vi "GymkhanaMonitoring.vi"() -> ()   [LabVIEW 2017]
uses:
  Control/GymkhanaBestIndicator(Monitoring).ctl
  Control/GymkhanaIndicator(Monitoring).ctl
  Control/GymkhanaData.ctl
panel:
  out "CurrentRecordIndicator":T1
  out "BestRecordIndicator":T2
  in  "Stop Button":bool
  # "2018 KSAE Formula Gymkhana Event"
  # "Time :"
  # "Time :"
  # "Entry :"
  # "Entry :"
  # "Univ. :"
  # "Univ. :"
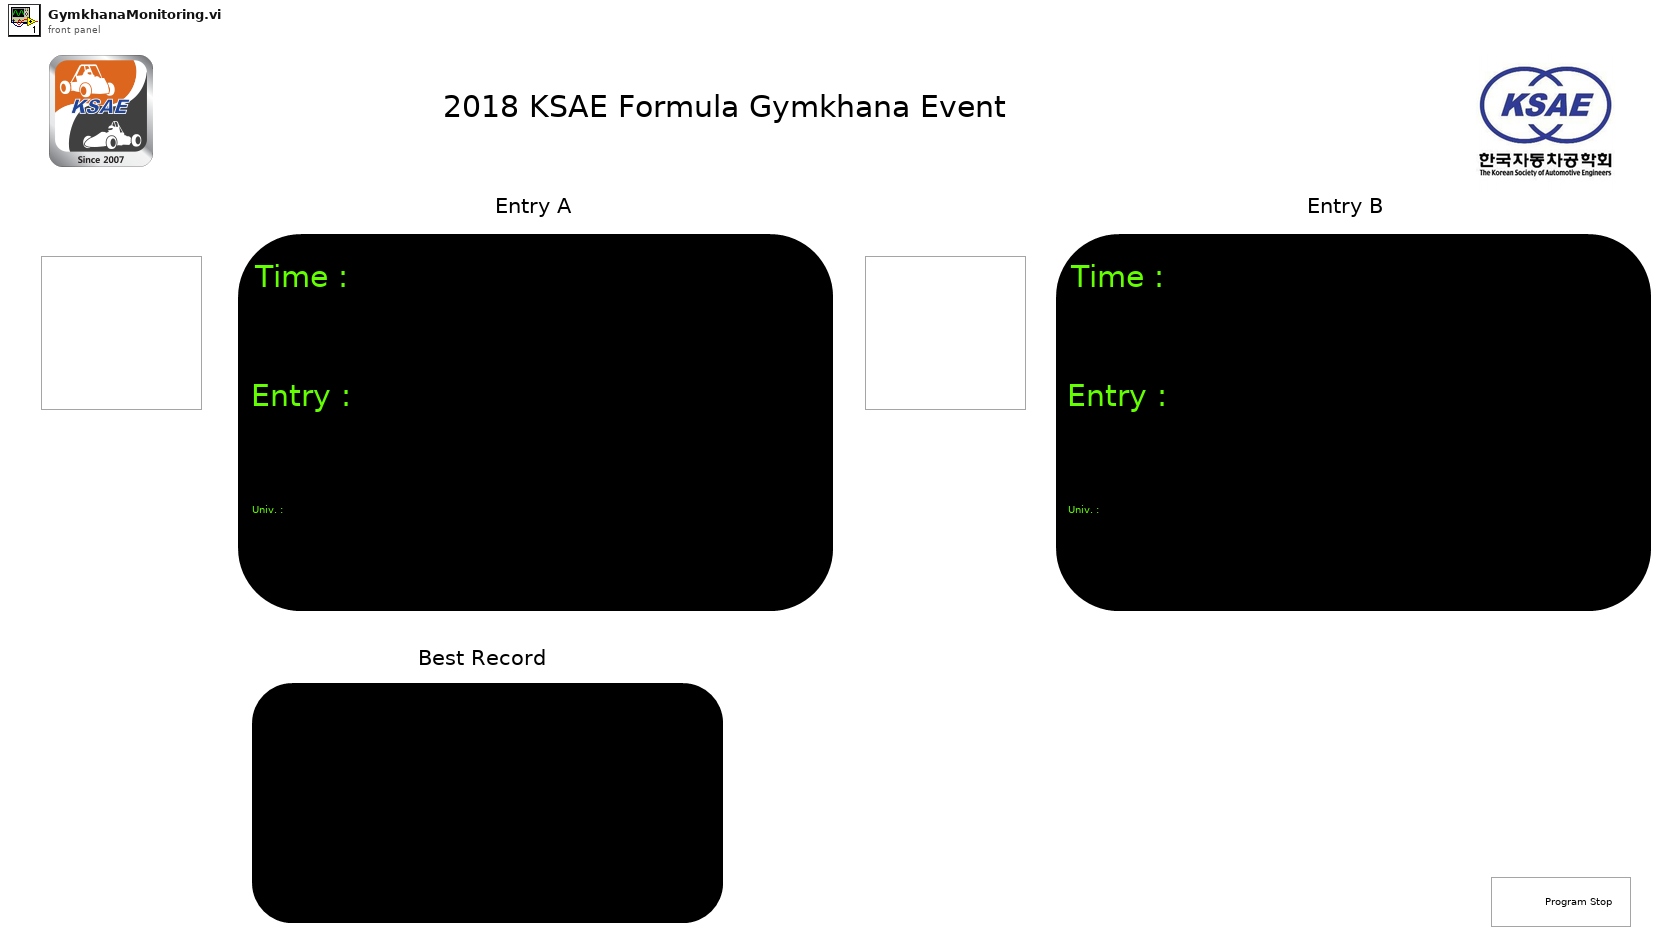
[diagram p1: front panel]
types:
  T1 = typedef "GymkhanaIndicator(Monitoring).ctl" = cluster{"CurrentTime-A":string, "CurrentEntry-A":string, "CurrentUniversity-A":string, "Flag-A":picture, "CurrentMessage-A":string, "CurrentTime-B":string, "CurrentEntry-B":string, "CurrentUniversity-B":string, "Flag-B":picture, "CurrentMessage-B":string}
  T2 = typedef "GymkhanaBestIndicator(Monitoring).ctl" = cluster{"BestTime":string, "BestEntry":string, "BestSchool":string}
  T3 = typedef "GymkhanaData.ctl" = cluster{"LabTime-A":string, "Entry-A":string, "University-A":string, "Flag-A":picture, "Message-A":string, "LabTime-B":string, "Entry-B":string, "University-B":string, "Flag-B":picture, "Message-B":string, "LabTime-Best":string, "Entry-Best":string, "University-Best":string}
  T4 = cluster{"Read Access":enum8{"Allowed", "Required", "None"}, "Write Access":enum8{"Allowed", "Required", "None"}}
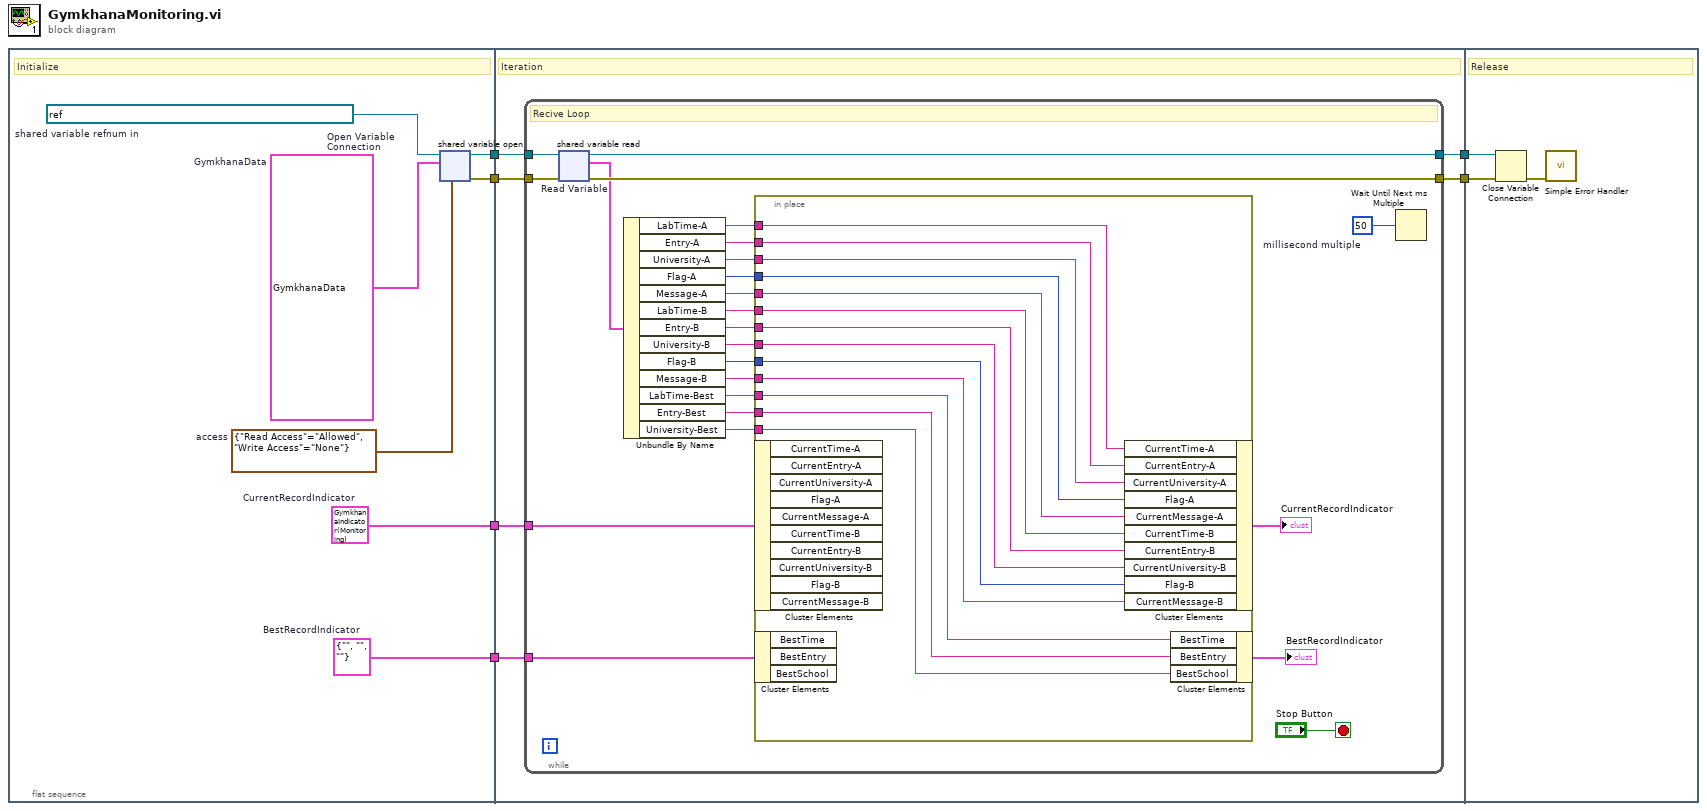
[diagram p0: block diagram]
diagram:
  n1 = flat-sequence {
    tunnel: [w13] -> w6
    tunnel: [w11] -> w5
    tunnel: [w8] -> w2
    tunnel: [w7] -> w1
    tunnel: w6 -> [w19]
    tunnel: w5 -> [w18]
    tunnel: [w17] -> w4
    tunnel: [w16] -> w3
    tunnel: w2 -> [w15]
    tunnel: w1 -> [w14]
    tunnel: w4 -> [w59]
    tunnel: w3 -> [w58]
    frame #0 {
      w7 = T2 {"BestTime"="", "BestEntry"="", "BestSchool"=""}  # BestRecordIndicator
      w8 = T1 {"CurrentTime-A"="", "CurrentEntry-A"="", "CurrentUniversity-A"="", "Flag-A"=bytes[0], "CurrentMessage-A"="", "CurrentTime-B"="", "CurrentEntry-B"="", "CurrentUniversity-B"="", "Flag-B"=bytes[0], "CurrentMessage-B"=""}  # CurrentRecordIndicator
      w9 = T3 {"LabTime-A"="", "Entry-A"="", "University-A"="", "Flag-A"=bytes[0], "Message-A"="", "LabTime-B"="", "Entry-B"="", "University-B"="", "Flag-B"=bytes[0], "Message-B"="", "LabTime-Best"="", "Entry-Best"="", "University-Best"=""}  # GymkhanaData
      w10 = refnum<k21> "ni.var.psp://kdh/MonitoringVariable/GymkhanaData"  # shared variable refnum in
      w12 = T4 {"Read Access"=enum."Allowed", "Write Access"=enum."None"}  # access
      # "Initialize"
      n2 = shared-variable-open "Open Variable Connection"(w10, w9, w12) -> (w13:refnum<k21>, w11:errorcluster)  [unwired: 1 in]
    }
    frame #1 {
      # "Iteration"
      n3 = while {
        tunnel: w19 -> [w43]
        tunnel: w18 -> [w42]
        tunnel: [w40] -> w16
        tunnel: [w39] -> w17
        tunnel: w15 -> [w37]
        tunnel: w14 -> [w24]
        stop <- "Stop Button" stop-if-true
        w41 = u32 50  # millisecond multiple
        # "Recive Loop"
        n4 = shared-variable-read "Read Variable"(w43, w42) -> (w40:refnum<k21>, w39:errorcluster, w38:T3)  [unwired: 1 out]
        n5 = Unbundle By Name(w38) -> ("LabTime-A"=w36:string, "Entry-A"=w35:string, "University-A"=w34:string, "Flag-A"=w33:picture, "Message-A"=w32:string, "LabTime-B"=w31:string, "Entry-B"=w30:string, "University-B"=w29:string, "Flag-B"=w28:picture, "Message-B"=w27:string, "LabTime-Best"=w22:string, "Entry-Best"=w21:string, "University-Best"=w20:string)
        n6 = in-place {
          in-place-border: w36 -> [w56]
          in-place-border: w35 -> [w55]
          in-place-border: w34 -> [w54]
          in-place-border: w33 -> [w53]
          in-place-border: w32 -> [w52]
          in-place-border: w31 -> [w47]
          in-place-border: w30 -> [w51]
          in-place-border: w29 -> [w50]
          in-place-border: w28 -> [w49]
          in-place-border: w27 -> [w48]
          in-place-border: w22 -> [w46]
          in-place-border: w21 -> [w45]
          in-place-border: w20 -> [w44]
          n7 = in-place-cluster #1(w37) -> ()  [unwired: 10 out]
          n8 = in-place-cluster #2(w24) -> ()  [unwired: 3 out]
          n9 = in-place-cluster #1("CurrentTime-A"=w56, "CurrentEntry-A"=w55, "CurrentUniversity-A"=w54, "Flag-A"=w53, "CurrentMessage-A"=w52, "CurrentTime-B"=w47, "CurrentEntry-B"=w51, "CurrentUniversity-B"=w50, "Flag-B"=w49, "CurrentMessage-B"=w48) -> (→"CurrentRecordIndicator":T1)
          n10 = in-place-cluster #2("BestTime"=w46, "BestEntry"=w45, "BestSchool"=w44) -> (→"BestRecordIndicator":T2)
        }
        n11 = Wait Until Next ms Multiple(millisecond multiple=w41) -> ()  [unwired: 1 out]
      }
    }
    frame #2 {
      # "Release"
      n12 = Close Variable Connection(8:w59, 11:w58) -> (0:w57:errorcluster)
      n13 = call <vilib>:"Simple Error Handler.vi"("error in (no error)"=w57) -> ()  [unwired: 4 in, 5 out]
    }
  }
